vi "Convert Data Status.vi"(8 "error in (no error)":errorcluster, 9 "Data Status String (\"\")":string, 11 "VISA resource name":refnum<visa-resource-name>) -> (0 "error out":errorcluster, 1 "Data Status":i32(ring) items=["Normal", "Differential Input", "Skip", "Over", "Error", "Burnout"], 3 "VISA resource name out":refnum<visa-resource-name>)   [LabVIEW 2020, in "Yokogawa GX Series.lvlib"]
doc: "This VI converts 1 character to a value as data status."
uses:
  <instrlib>/Yokogawa GX Series/Yokogawa GX Series.lvlib
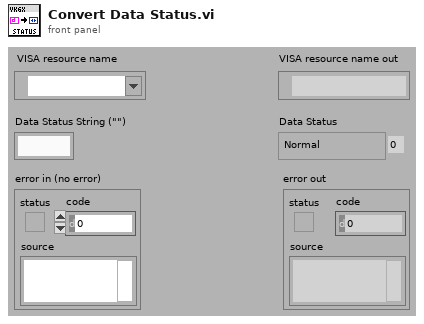
[diagram p1: front panel]
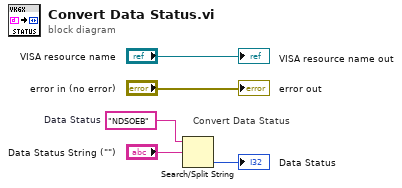
[diagram p0: block diagram]
diagram:
  w2 = "NDSOEB"  # Data Status
  # "Convert Data Status"
  n1 = Search/Split String(string=w2, search string/char (-)="Data Status String (\"\")") -> (offset of match=→"Data Status":i32)  [unwired: 3 out]
  "VISA resource name out" <- "VISA resource name"
  "error out" <- "error in (no error)"
